vi "CALC_FILT_GATE_TIME_SPAN.vi"(0 "VISA IN":refnum<visa-resource-name>, 1 "Time Span(sec)":i32, 5 "error in":errorcluster, 7 "Channel":i32) -> (14 "VISA Out":refnum<visa-resource-name>, 19 "error out":errorcluster)   [LabVIEW 2018, in "PNA-X.lvlib"]
doc: "CALCulate<cnum>:FILTer[:GATE]:TIME:SPAN <num> \n(Read-Write) Sets the gate filter span time. \nSee Critical Note \nParameters \n<cnum> Channel number of the measurement. There must be a selected measurement \non that channel. If unspecified, <cnum> is set to 1. \n<num> Time span in seconds; Choose any number between: \n0 and 2* [(number of points-1) / frequency span] \nNote: This command will accept MIN or MAX instead of a numeric \nparameter. See SCPI Syntax for more information. \nExamples CALC:FILT:GATE:TIME:SPAN 5 ns \ncalculate2:filter:time:span maximum \nQuery Syntax CALCulate<cnum>:FILTer[:GATE]:TIME:SPAN? \nReturn Type Numeric \nDefault 20 ns"
uses:
  PNA-X.lvlib
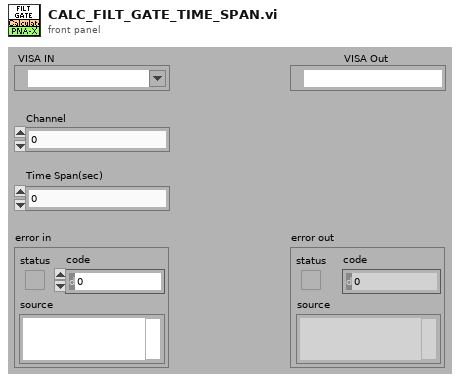
[diagram p1: front panel]
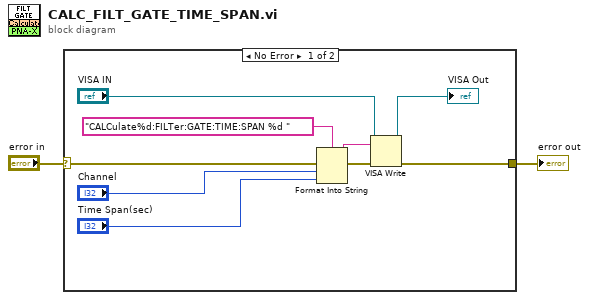
[diagram p0: block diagram]
diagram:
  n1 = case shown="No Error" "error in" {
    selector: "error in" -> [w11 w12]
    tunnel: [w6 w12] -> w1
    frame No Error {
      n2 = Format Into String(format string="CALCulate%d:FILTer:GATE:TIME:SPAN %d " ("Cmdline"), error in=w11, "Channel", "Time Span(sec)") -> (resulting string=w9:string, error out=w10:errorcluster)  [unwired: 1 in]
      n3 = VISA Write(VISA resource name="VISA IN", write buffer=w9, error in (no error)=w10) -> (VISA resource name out=→"VISA Out":refnum<visa-resource-name>, error out=w6:errorcluster)  [unwired: 1 out]
    }
    frame Error {
    }
  }
  "error out" <- w1
